vi "EOL CAN_Get_Motor_SW_CAL_Boot_Level.vi"(7 "Rx Arbitration Id":u32=402522244 format="%.0x", 8 "error in (no error)":errorcluster, 9 "Tx Arbitration Id":u32=402391172 format="%.0x", 10 "Read Session in":refnum<k21>, 11 "Write Session in":refnum<k21>) -> (0 "error out":errorcluster, 1 "CAL level":string, 2 "Boot level":string, 3 "SW level":string, 4 "Response Good?":bool, 5 "TxRx Data":string[][](array[string]))   [LabVIEW 2014]
uses:
  <vilib>/xnet/xnet.llb/XNET Frame CAN.ctl
  <vilib>/xnet/xnet.llb/XNET Frame Type CAN.ctl
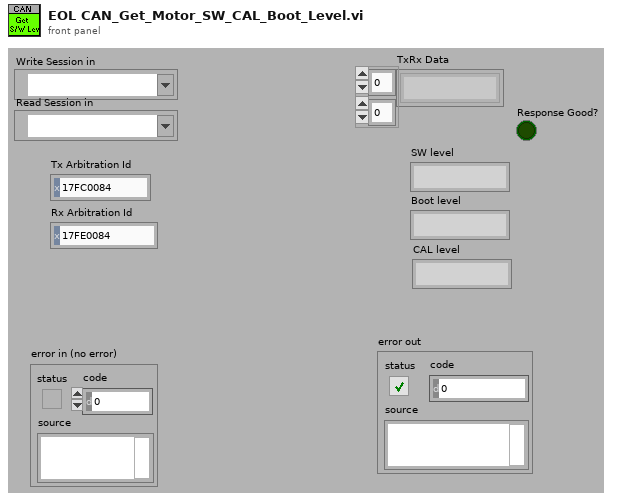
[diagram p1: front panel]
types:
  T1 = typedef "XNET Frame CAN.ctl" = cluster{"timestamp":timestamp, "payload":u8[], "identifier":u32, "type":T2, "extended?":bool, "echo?":bool}
  T2 = typedef "XNET Frame Type CAN.ctl" = u8
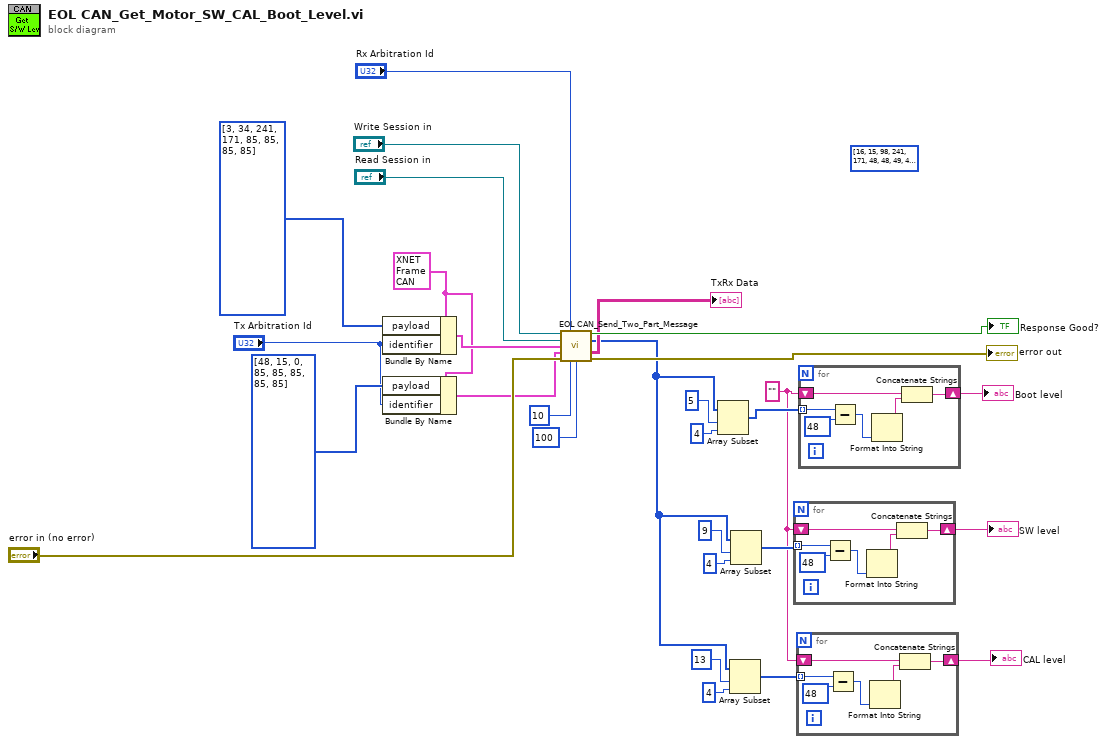
[diagram p0: block diagram]
diagram:
  w6 = T1 {"timestamp"=timestamp(0 s since 1904-01-01), "payload"=[2, 39, 3, 85, 85, 85, 85, 85], "identifier"=402391172, "type"=0, "extended?"=TRUE, "echo?"=FALSE} ("Tx CAN frame 1")
  (unwired) u8[] [16, 15, 98, 241, 171, 48, 48, 49, 48, 48, 48, 48, 53, 48, 48, 48, 51, 170, 170, 170, 170, 170] ("Rx Data")
  w13 = ""
  n1 = Bundle By Name(cluster=w6, "payload"=u8[] [3, 34, 241, 171, 85, 85, 85, 85] ("Transmit Data"), "identifier"="Tx Arbitration Id") -> (w7:T1)
  n2 = Bundle By Name(cluster=w6, "payload"=u8[] [48, 15, 0, 85, 85, 85, 85, 85] ("Transmit Data"), "identifier"="Tx Arbitration Id") -> (w5:T1)
  n3 = call "EOL CAN_Send_Two_Part_Message.vi"("Write Session in"="Write Session in", "Rx Arbitration Id"="Rx Arbitration Id", "Read Session in"="Read Session in", "Tx CAN frame 1"=w7, "Tx CAN frame 2"=w5, "error in (no error)"="error in (no error)", "Retries"=10, "Msg Wait Time"=u32 100) -> ("Response Good?"=→"Response Good?":bool, "Rx Data"=w12:u8[], "TxRx Data"=→"TxRx Data":string[][], "error out"=→"error out":errorcluster)  [unwired: 4 in]
  n4 = Array Subset(array=w12, index=5, length=4) -> (w18:u8[])
  n5 = Array Subset(array=w12, index=13, length=4) -> (w16:u8[])
  n6 = Array Subset(array=w12, index=9, length=4) -> (w17:u8[])
  n7 = for {
    shift-right: [w34] -> w15
    shift-left: w13 -> [w33]
    tunnel: w17 -> [w32] mode=indexing
    n8 = Subtract(x=w32, y=u8 48) -> (x-y=w30:u8)
    n9 = Format Into String(w30) -> (resulting string=w35:string)  [unwired: 3 in, 1 out]
    n10 = Concatenate Strings(w33, w35) -> (w34:string)
  }
  "SW level" <- w15
  n11 = for {
    shift-right: [w40] -> w14
    shift-left: w13 -> [w39]
    tunnel: w16 -> [w38] mode=indexing
    n12 = Subtract(x=w38, y=u8 48) -> (x-y=w36:u8)
    n13 = Format Into String(w36) -> (resulting string=w41:string)  [unwired: 3 in, 1 out]
    n14 = Concatenate Strings(w39, w41) -> (w40:string)
  }
  "CAL level" <- w14
  n15 = for {
    shift-right: [w46] -> w21
    shift-left: w13 -> [w45]
    tunnel: w18 -> [w44] mode=indexing
    n16 = Subtract(x=w44, y=u8 48) -> (x-y=w42:u8)
    n17 = Format Into String(w42) -> (resulting string=w47:string)  [unwired: 3 in, 1 out]
    n18 = Concatenate Strings(w45, w47) -> (w46:string)
  }
  "Boot level" <- w21
